vi "Get Config File Sections.vi"(8 "error in (no error)":errorcluster, 11 "Configuration File in":refnum<class "Configuration File.lvclass">) -> (0 "error out":errorcluster, 2 "Section names":string[](array[string]), 3 "Configuration File out":refnum<class "Configuration File.lvclass">)   [LabVIEW 2018, in "Configuration File.lvlib" / "Configuration File.lvclass"]
doc: "This method reads all the sections from the configuration file and returns an array with them."
uses:
  Configuration File.lvclass
  Configuration File.lvclass/Configuration File.ctl
  <vilib>/Utility/config.llb/NI_LVConfig.lvlib
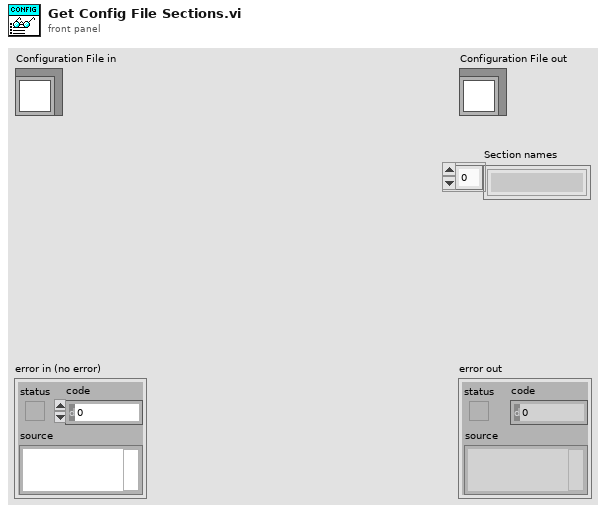
[diagram p1: front panel]
types:
  T1 = typedef "NI_LVConfig.lvlib/Config Data RefNum.ctl" = refnum<k1>
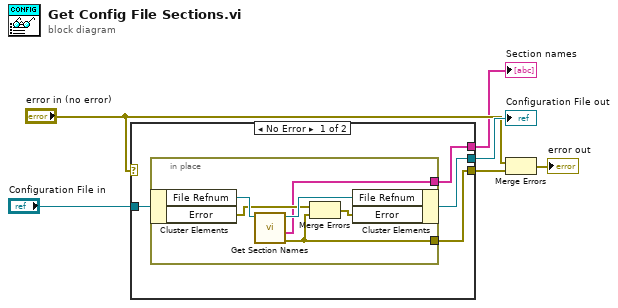
[diagram p0: block diagram]
diagram:
  n1 = case shown="No Error" "error in (no error)" {
    selector: "error in (no error)" -> [_ w18]
    tunnel: [w8 w18] -> w6
    tunnel: [w9 w17] -> w4
    tunnel: "Configuration File in" -> [w10 w17]
    tunnel: [w7 _] -> w1
    frame No Error {
      n2 = in-place {
        in-place-border: [w14] -> w8
        in-place-border: [w11] -> w7
        n3 = in-place-cluster #1(w10) -> ("File Refnum"=w16:T1, "Error"=w12:errorcluster)
        n4 = call <vilib>:"Get Section Names.vi"("refnum"=w16) -> ("error out"=w14:errorcluster, "section names"=w11:string[], "refnum out"=w15:T1)  [unwired: 8 in]
        n5 = Merge Errors(w12, w14) -> (w13:errorcluster)
        n6 = in-place-cluster #1("File Refnum"=w15, "Error"=w13) -> (w9:refnum<class "Configuration File.lvclass">)
      }
    }
    frame Error {
    }
  }
  "Configuration File out" <- w4
  "Section names" <- w1
  n7 = Merge Errors("error in (no error)", w6) -> (→"error out":errorcluster)
